vi "Write Color.vi"(10 "Color":T1, 11 "Piece in":refnum<class "Piece.lvclass">) -> (3 "Piece out":refnum<class "Piece.lvclass">)   [LabVIEW 2015, in "Chesslib.lvlib" / "Piece.lvclass"]
uses:
  Piece.lvclass
  typedef/Color.ctl
  Piece.lvclass/Piece.ctl
  Chesslib.lvlib
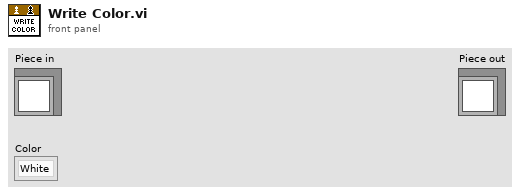
[diagram p1: front panel]
types:
  T1 = typedef "Chesslib.lvlib/Color.ctl" = enum16{"White", "Black"}
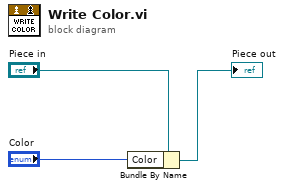
[diagram p0: block diagram]
diagram:
  n1 = Bundle By Name(cluster="Piece in", "Color"="Color") -> (→"Piece out":refnum<class "Piece.lvclass">)
